vi "设置定时时间.vi"(8 "error in (no error)":errorcluster caption="错误输入（无错误）", 9 "设置时间":u32, 11 "定时器类 输入":refnum<class "定时器类.lvclass">) -> (0 "error out":errorcluster caption="错误输出", 3 "定时器类 输出":refnum<class "定时器类.lvclass">)   [LabVIEW 2014, in "定时器类.lvclass"]
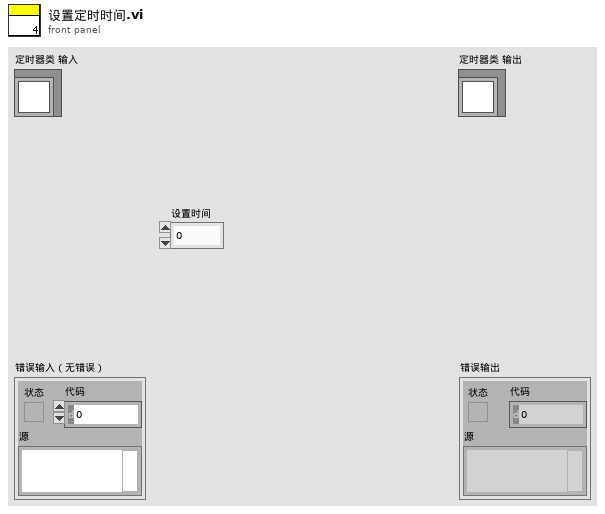
[diagram p1: front panel]
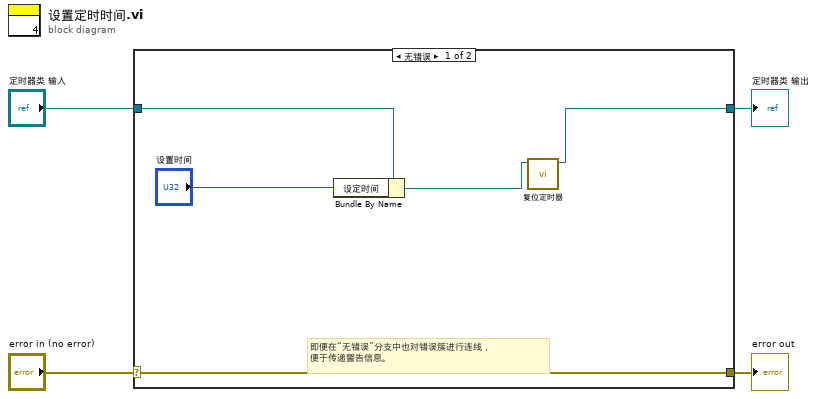
[diagram p0: block diagram]
diagram:
  n1 = case shown="无错误" "error in (no error)" {
    selector: "error in (no error)" -> [w9 w11]
    tunnel: [w9 w11] -> w3
    tunnel: [w5 w10] -> w1
    tunnel: "定时器类 输入" -> [w7 w10]
    frame No Error {
      # "即便在“无错误”分支中也对错误簇进行连线，\n便于传递警告信息。"
      n2 = Bundle By Name(cluster=w7, "设定时间"="设置时间") -> (w6:refnum<class "定时器类.lvclass">)
      n3 = call-dynamic "复位定时器.vi"("定时器类 输入"=w6) -> ("定时器类 输出"=w5:refnum<class "定时器类.lvclass">)  [unwired: 9 in, 1 out]
    }
    frame Error {
    }
  }
  "error out" <- w3
  "定时器类 输出" <- w1
